vi "Digital Write Pin.vi"(8 "Error In":errorcluster, 9 "Value (Off)":bool, 10 "Digital I/O Pin (2)":u8=2, 11 "ChipKit Resource":T1={"COM Port"="", "Board Type"=enum."ChipKit Uno32", "Connection Type"=enum."USB / Serial", "Baud Rate (115200)"=115200, "Bytes Per Packet (15)"=15}) -> (0 "Error Out":errorcluster, 3 "ChipKit Resource":T1={"COM Port"="", "Board Type"=enum."ChipKit Uno32", "Connection Type"=enum."USB / Serial", "Baud Rate (115200)"=115200, "Bytes Per Packet (15)"=15})   [LabVIEW 2011, in "LabVIEW Interface for ChipKit.lvlib"]
doc: "Writes the specified value on the selected digital output pin (D0 - D13). The pin must fist be configured as an output using the ChipKit Set Digital Pin Mode VI."
uses:
  LabVIEW Interface for ChipKit.lvlib
  Private/Type Defs/Chipkit Resource.ctl
  Private/Type Defs/Board Type.ctl
  Private/Type Defs/Connection Type.ctl
  Private/Type Defs/Command.ctl
  Private/Type Defs/Pin Type.ctl
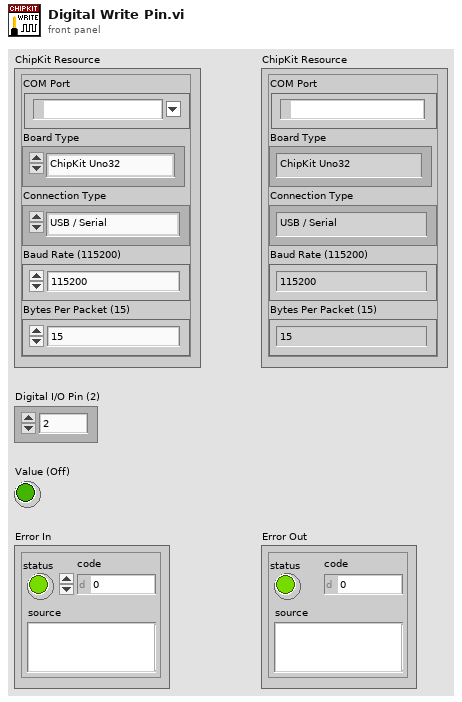
[diagram p1: front panel]
types:
  T1 = typedef "LabVIEW Interface for ChipKit.lvlib/Chipkit Resource.ctl" = cluster{"COM Port":refnum<visa-resource-name>, "Board Type":T2, "Connection Type":T3, "Baud Rate (115200)":u32, "Bytes Per Packet (15)":u32}
  T2 = typedef "LabVIEW Interface for ChipKit.lvlib/Board Type.ctl" = enum16{"ChipKit uC32", "ChipKit Uno32", "ChipKit Max32"}
  T3 = typedef "LabVIEW Interface for ChipKit.lvlib/Connection Type.ctl" = enum8{"USB / Serial", "XBEE", "BlueSmirf (Bluetooth)"}
  T4 = typedef "LabVIEW Interface for ChipKit.lvlib/Pin Type.ctl" = enum8{"Analog", "Digital", "PWM", "Tone"}
  T5 = typedef "LabVIEW Interface for ChipKit.lvlib/Command.ctl" = enum8{"setArduinoMode", "flushSerial", "setPinMode", "digitalWritePin", "digitalWritePort", "tone", "digitalReadPin", "digitalReadPort", "analogReadPin", "analogReadPort", "pwmWritePin", "pwmWritePort", "sevenSegment_Configure", "sevenSegment_Write", "I2C Init", "I2C Write", "I2C Read", "SPI Init", "SPI Set Bit Order", "SPI Set Clock Divider", "SPI Set Data Mode", "SPI Send / Receive", "SPI Close", "Servo Set Num Servos", "Servo Config Servo", "Servo Write Angle", "Servo Read Angle", "Servo Write Pulse Width", "Servo Read Pulse Width", "Servo Detach", "LCD Init", "LCD Set Size", "LCD Set Cursor Mode", "LCD Clear", "LCD Set Cursor Position", "LCD Print", "LCD Display Power", "LCD Scroll Display", "LCD Autoscroll", "LCD Print Direction", "LCD Create Custom Char", "LCD Print Custom Char", "contAcqOn", "contAcqOff", "getFirmwareVersion", "FiniteSampleStart"}
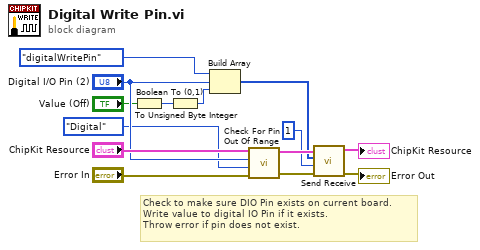
[diagram p0: block diagram]
diagram:
  # "Check to make sure DIO Pin exists on current board.\nWrite value to digital IO Pin if it exists.\nThrow error if pin does not exist."
  n1 = Boolean To (0,1)(Boolean="Value (Off)") -> (0, 1=w3:i16)
  n2 = To Unsigned Byte Integer(number=w3) -> (unsigned 8bit integer=w2:u8)
  n3 = Build Array(Command."digitalWritePin" ("Command"), "Digital I/O Pin (2)", w2) -> (w6:u8[])
  n4 = call "Check For Pin Out Of Range.vi"("Error In"="Error In", "Pin Type"=Pin_Type."Digital", "User Pin Number"="Digital I/O Pin (2)", "Arduino Resource"="ChipKit Resource") -> ("Error Out"=w7:errorcluster, "Arduino Resource"=w10:T1)  [unwired: 6 in]
  n5 = call "Send Receive.vi"("Error In"=w7, "Bytes To Read (0)"=u32 1, "Data"=w6, "ChipKit Resource"=w10) -> ("Error Out"=→"Error Out":errorcluster, "ChipKit Resource"=→"ChipKit Resource":T1)  [unwired: 5 in, 1 out]
